vi "Read Status.vi"(8 "error in":errorcluster, 11 "3022A in":refnum<class "3022A.lvclass">) -> (0 "error out":errorcluster, 2 "Ready?":bool, 3 "3022A out":refnum<class "3022A.lvclass">)   [LabVIEW 2014, in "3022A.lvclass"]
uses:
  3022A.lvclass
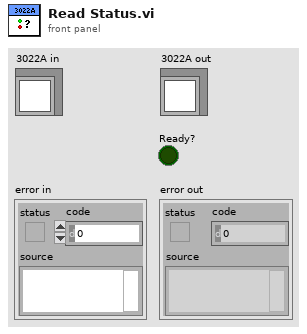
[diagram p1: front panel]
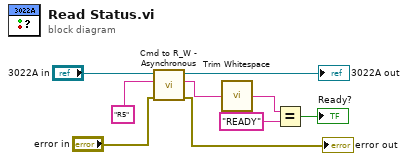
[diagram p0: block diagram]
diagram:
  n1 = call-dynamic "Cmd to R_W - Asynchronous.vi"("error in"="error in", "write buffer"="R5" ("string"), "Serial IO in"="3022A in") -> ("error out"=→"error out":errorcluster, "read buffer"=w4:string, "Serial IO out"=→"3022A out":refnum<class "3022A.lvclass">)  [unwired: 6 in]
  n2 = call <vilib>:"Trim Whitespace.vi"("string"=w4) -> ("trimmed string"=w3:string)  [unwired: 1 in]
  n3 = Equal?(x=w3, y="READY") -> (x = y?=→"Ready?":bool)
